vi "Msg - FP Elt - (N) Update Values.vi"(0 "Messages":T1[](array[typedef]), 11 "error in (no error)":errorcluster) -> (15 "error out":errorcluster)   [LabVIEW 2016, in "Template.lvlib"]
doc: "Send (N) Messages to this Module to update the value of certain of its FP Elements."
uses:
  Template.lvlib
  Controls/FP - Update Value.ctl
  Controls/FP - Actionable Element.ctl
  Controls/Message.ctl
  Controls/Module - States.ctl
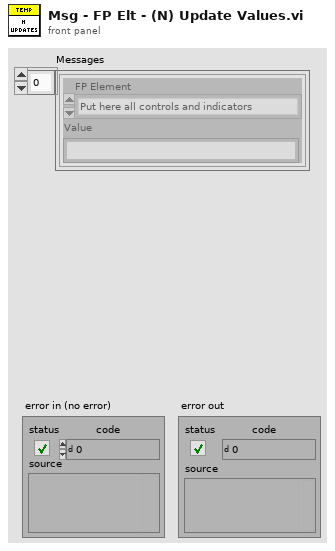
[diagram p1: front panel]
types:
  T1 = typedef "Template.lvlib/FP - Update Value.ctl" = cluster{"FP Element":T2, "Value":string}
  T2 = typedef "Template.lvlib/FP - Actionable Element.ctl" = enum16{"Put here all controls and indicators", "belonging to the UI of this module", "whose value can ", "be updated programatically", "or which can be enabled or disabled", ""}
  T3 = typedef "Template.lvlib/Message.ctl" = cluster{"State":T4, "Data":variant, "Transitioning State?":bool}
  T4 = typedef "Template.lvlib/Module - States.ctl" = enum16{"Initialize", "Event ", "Send data", "FP Element: Update", "FP Element: Disable/Enable", "Timer: Setup", "Terminate", "---------------Template---------------"}
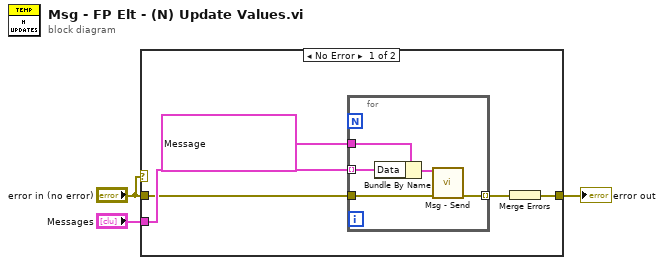
[diagram p0: block diagram]
diagram:
  n1 = case shown="No Error" "error in (no error)" {
    tunnel: [w4 w14] -> w3
    tunnel: "error in (no error)" -> [w6 w14]
    tunnel: "Messages" -> [w8 _]
    frame No Error {
      n2 = for {
        tunnel: w8 -> [w13] mode=indexing
        tunnel: T3 {"State"=enum."FP Element: Update", "Data"=variant, "Transitioning State?"=FALSE} ("Message") -> [w12]
        tunnel: w6 -> [w10]
        tunnel: [w9] -> w5 mode=indexing
        n3 = Bundle By Name(cluster=w12, "Data"=w13) -> (w11:T3)
        n4 = call "Msg - Send.vi"("Message"=w11, "error in (no error)"=w10) -> ("error out"=w9:errorcluster)  [unwired: 13 in]
      }
      n5 = Merge Errors(w5) -> (w4:errorcluster)
    }
    frame Error {
    }
  }
  "error out" <- w3
